vi "Read Time.vi"(8 "error in (no error)":errorcluster, 11 "ControlKeyUpMsg in":refnum<class "ControlKeyUpMsg.lvclass">) -> (0 "error out":errorcluster, 2 "Time":u32, 3 "ControlKeyUpMsg out":refnum<class "ControlKeyUpMsg.lvclass">)   [LabVIEW 2015, in "ActorEvents.lvlib" / "ControlKeyUpMsg.lvclass"]
uses:
  ControlKeyUpMsg.lvclass
  ControlKeyUpMsg.lvclass/ControlKeyUpMsg.ctl
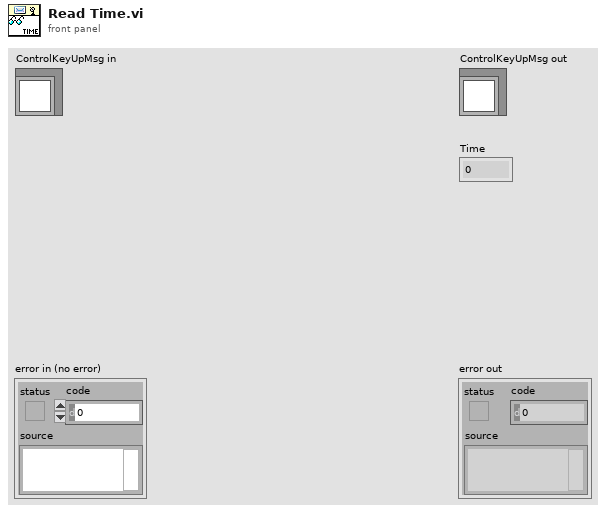
[diagram p1: front panel]
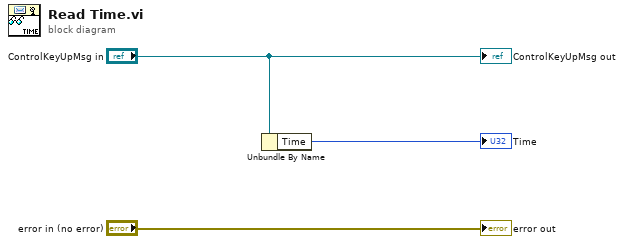
[diagram p0: block diagram]
diagram:
  n1 = Unbundle By Name("ControlKeyUpMsg in") -> ("Time"=→"Time":u32)
  "error out" <- "error in (no error)"
  "ControlKeyUpMsg out" <- "ControlKeyUpMsg in"
